vi "oa_Search Start and End in Speed Profile (Speed).vi"(6 "last value in":cluster{"reference":dbl, "interpolation":dbl}, 7 "reset":bool, 8 "steps input":cluster{"start":dbl, "end":dbl, "step":dbl} {"step" format="%.2f"; "end" format="%.2f"; "start" format="%.2f"}, 9 "next value in":dbl, 10 "interpolation array":dbl[](array[numeric]), 11 "reference array":dbl[](array[numeric])) -> (0 "actual steps":T1 {"step" format="%.2f"; "start" format="%.2f"}, 1 "next value out":dbl, 2 "interpolation array out":dbl[](array[numeric]), 3 "reference array out":dbl[](array[numeric]), 4 "last value out":cluster{"reference":dbl, "interpolation":dbl}, 5 "reach end?":bool)   [LabVIEW 2017]
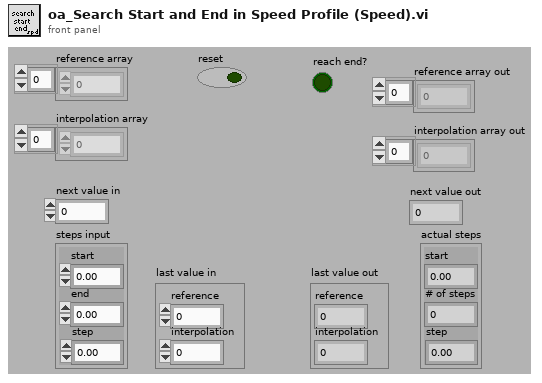
[diagram p1: front panel]
types:
  T1 = cluster{"start":dbl, "# of steps":i32, "step":dbl}
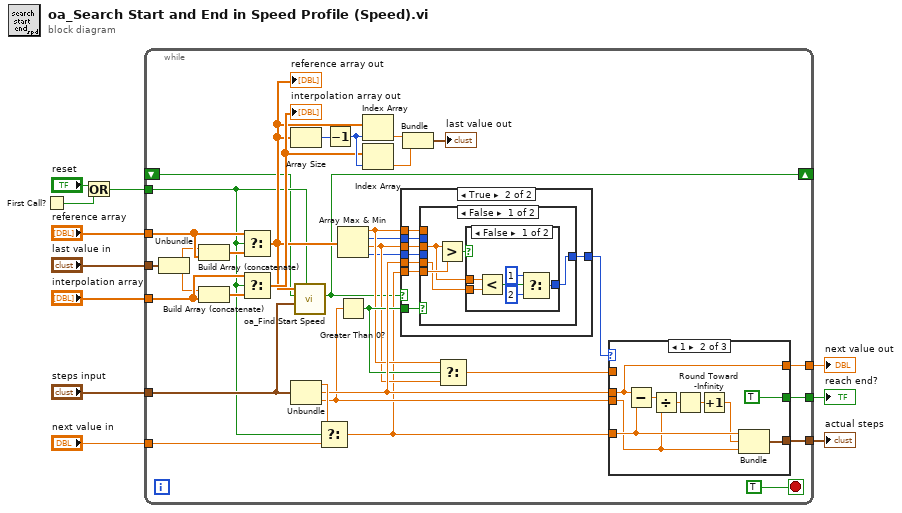
[diagram p0: block diagram]
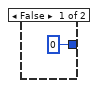
[diagram p2: hidden frame]
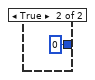
[diagram p3: hidden frame]
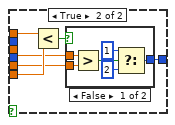
[diagram p4: hidden frame]
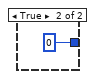
[diagram p5: hidden frame]
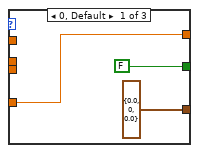
[diagram p6: hidden frame]
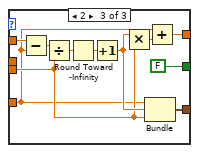
[diagram p7: hidden frame]
diagram:
  n1 = First Call?() -> (First Call?: T/F=w10:bool)
  n2 = Or(x="reset", y=w10) -> (x .or. y?=w1:bool)
  n3 = while {
    tunnel: "next value in" -> [w45]
    tunnel: "last value in" -> [w44]
    tunnel: "reference array" -> [w43]
    tunnel: "interpolation array" -> [w42]
    tunnel: [w41] -> w5
    tunnel: [w40] -> w4
    tunnel: [w39] -> w3
    tunnel: "steps input" -> [w17]
    tunnel: w1 -> [w15]
    shift-right: [w12] -> _
    shift-left: _ -> [w13]
    stop <- TRUE stop-if-true
    n4 = Unbundle(w44) -> ("reference"=w37:dbl, "interpolation"=w34:dbl)
    n5 = Build Array (concatenate)(w37, w43) -> (w36:dbl[])
    n6 = Build Array (concatenate)(w34, w42) -> (w35:dbl[])
    n7 = Select(t=w43, s=w15, f=w36) -> (s? t:f=w16:dbl[])
    "reference array out" <- w16
    n8 = Select(t=w42, s=w15, f=w35) -> (s? t:f=w20:dbl[])
    "interpolation array out" <- w20
    n9 = Array Size(array=w16) -> (size(s)=w33:i32)
    n10 = Unbundle(w17) -> ("start"=w38:dbl, "end"=w28:dbl, "step"=w23:dbl)
    n11 = call <vilib>:"oa_Find Start Speed.vi"("reset"=w15, "steps input"=w17, "start found"=w13, "reference array"=w16) -> ("find start?"=w12:bool)  [unwired: 7 in]
    n12 = Select(t=w38, s=w15, f=w45) -> (s? t:f=w18:dbl)
    n13 = Decrement(x=w33) -> (x-1=w32:i32)
    n14 = Array Max & Min(array=w16) -> (max value=w26:dbl, max index (indices)=w22:i32, min value=w25:dbl, min index (indices)=w21:i32)
    n15 = Greater Than 0?(x=w23) -> (x > 0?=w27:bool)
    n16 = Index Array(array=w16, index=w32) -> (element=w31:dbl)
    n17 = Index Array(array=w20, index=w32) -> (element=w30:dbl)
    n18 = case shown="True" w12 {
      tunnel: w28 -> [_ w54]
      tunnel: w27 -> [_ w53]
      tunnel: w26 -> [_ w52]
      tunnel: w25 -> [_ w51]
      tunnel: w22 -> [_ w50]
      tunnel: w21 -> [_ w49]
      tunnel: [0 ("f") w48] -> w19
      tunnel: w18 -> [_ w47]
      frame False {
      }
      frame True {
        n19 = case shown="False" w53 {
          tunnel: w52 -> [_ w68]
          tunnel: w51 -> [w56 _]
          tunnel: w47 -> [w59 w71]
          tunnel: w54 -> [w57 w70]
          tunnel: [w58 w69] -> w48
          tunnel: w50 -> [_ _]
          tunnel: w49 -> [_ _]
          frame False {
            n20 = Greater?(x=w56, y=w59) -> (0:w55:bool)
            n21 = case shown="False" w55 {
              tunnel: [w61 0] -> w58
              tunnel: w56 -> [w65 _]
              tunnel: w57 -> [w64 _]
              frame False {
                n22 = Less?(x=w65, y=w64) -> (x < y?=w63:bool)
                n23 = Select(t=1, s=w63, f=2) -> (s? t:f=w61:i32)
              }
              frame True {
              }
            }
          }
          frame True {
            n24 = Less?(x=w68, y=w71) -> (x < y?=w67:bool)
            n25 = case shown="False" w67 {
              tunnel: w68 -> [w77 _]
              tunnel: w70 -> [w76 _]
              tunnel: [w72 0] -> w69
              frame False {
                n26 = Greater?(x=w77, y=w76) -> (0:w75:bool)
                n27 = Select(t=1, s=w75, f=2) -> (s? t:f=w72:i32)
              }
              frame True {
              }
            }
          }
        }
      }
    }
    n28 = Bundle("time [s]"=w31, "speed [rpm]"=w30) -> (→"last value out":cluster{"time [s]":dbl, "speed [rpm]":dbl})  [unwired: 1 in]
    n29 = Select(t=w26, s=w27, f=w25) -> (s? t:f=w24:dbl)
    n30 = case shown="1" w19 {
      tunnel: [FALSE ("reach end?") TRUE ("reach end?") FALSE ("reach end?")] -> w41
      tunnel: w18 -> [w80 w89 w93]
      tunnel: [w80 w84 w95] -> w40
      tunnel: [T1 {"start"=0.0, "# of steps"=0, "step"=0.0} ("actual steps") w85 w99] -> w39
      tunnel: w23 -> [_ w87 w97]
      tunnel: w28 -> [_ w84 _]
      tunnel: w24 -> [_ _ w94]
      frame 0, Default {
      }
      frame 1 {
        n31 = Subtract(x=w84, y=w89) -> (x-y=w88:dbl)
        n32 = Divide(x=w88, y=w87) -> (x/y=w83:dbl)
        n33 = Round Toward -Infinity(1:w83) -> (0:w82:dbl)
        n34 = Increment(x=w82) -> (x+1=w86:dbl)
        n35 = Bundle("next value in"=w89, w86, "step"=w87) -> (w85:cluster{"next value in":dbl, dbl, "step":dbl})  [unwired: 1 in]
      }
      frame 2 {
        n36 = Subtract(x=w94, y=w93) -> (x-y=w100:dbl)
        n37 = Divide(x=w100, y=w97) -> (x/y=w92:dbl)
        n38 = Round Toward -Infinity(1:w92) -> (0:w91:dbl)
        n39 = Increment(x=w91) -> (x+1=w98:dbl)
        n40 = Multiply(x=w98, y=w97) -> (x*y=w96:dbl)
        n41 = Bundle("next value in"=w93, w98, "step"=w97) -> (w99:cluster{"next value in":dbl, dbl, "step":dbl})  [unwired: 1 in]
        n42 = Add(x=w93, y=w96) -> (x+y=w95:dbl)
      }
    }
  }
  "next value out" <- w4
  "reach end?" <- w5
  "actual steps" <- w3
